vi "Change Qpurge.vi"(8 "error in":errorcluster, 11 "tCRD in":refnum<class "Open Path CRD.lvclass">) -> (0 "error out":errorcluster, 3 "tCRD out":refnum<class "Open Path CRD.lvclass">)   [LabVIEW 2015, in "Open Path CRD.lvclass"]
uses:
  Open Path CRD.lvclass
  Reusable/Instrument/Instrument.lvclass/Instrument.ctl
  Open Path CRD.lvclass/Open Path CRD.ctl
  Reusable/Instrument/Read Log Session.vi
  Reusable/CRDS/Main/Read Data.vi
  Reusable/CRDS/Data/Main/Read filter.vi
  Reusable/CRDS/Data/Main/CRDS Data.lvclass
  <userlib>/_Session Fwk/Session - Root.lvclass
  Devices/Alicat/Session Based/Alicat Device.lvclass
  Reusable/Session Log/System Log.lvclass
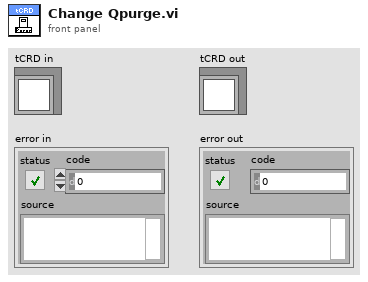
[diagram p1: front panel]
types:
  T1 = typedef "Session - Root.lvclass/Session Handle.ctl" = refnum<data-value>
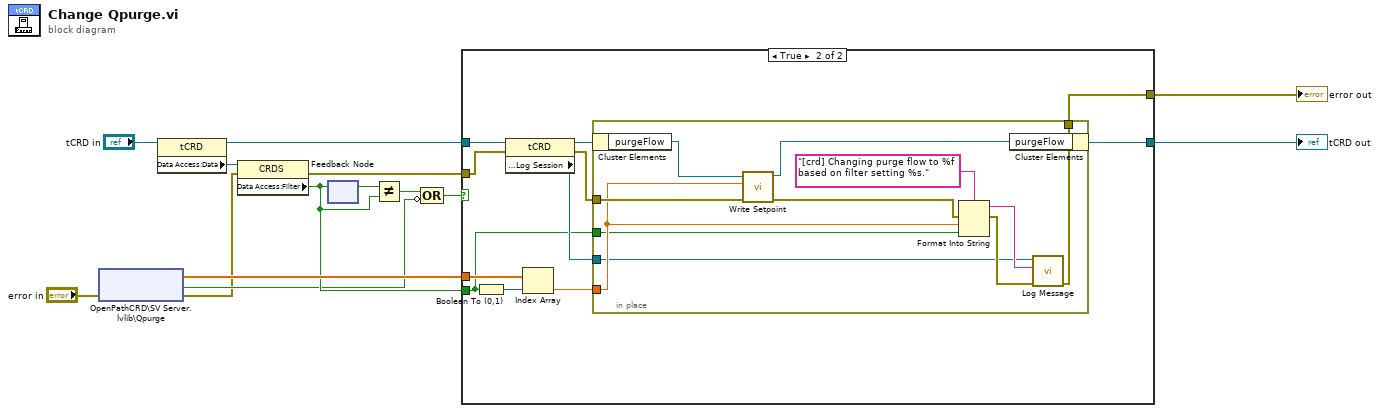
[diagram p0: block diagram]
diagram:
  n1 = shared-variable "OpenPathCRD\\SV Server.lvlib\\Qpurge"(error in="error in") -> (w11:sgl[], error out=w2:errorcluster, w3:bool)  [unwired: 1 in]
  n2 = property class="tCRD"(reference="tCRD in") -> (reference out=w9:refnum<class "Open Path CRD.lvclass">, "Data Access:Data"=w8:refnum<class "CRDS Data.lvclass">)  [unwired: 1 in, 1 out]
  n3 = property class="CRDS"(reference=w8, error in=w2) -> (error out=w1:errorcluster, "Data Access:Filter"=w4:bool)  [unwired: 1 out]
  n4 = feedback-in #1(w4) -> ()
  n5 = feedback #1() -> (w7:bool)  [unwired: 1 in]
  n6 = Not Equal?(x=w7, y=w4) -> (x != y?=w6:bool)
  n7 = Compound Arithmetic op=OR(w6, invert w3) -> (w5:bool)
  n8 = case shown="True" w5 {
    tunnel: w9 -> [w16 w26]
    tunnel: [w16 w27] -> w12
    tunnel: [w15 w24] -> w14
    tunnel: w11 -> [_ w22]
    tunnel: w4 -> [_ w20]
    tunnel: w1 -> [w15 w17]
    frame False {
    }
    frame True {
      n9 = Boolean To (0,1)(Boolean=w20) -> (0, 1=w23:i16)
      n10 = property class="tCRD"(reference=w26, error in=w17) -> (reference out=w19:refnum<class "Open Path CRD.lvclass">, error out=w18:errorcluster, "Accessors:Log Session"=w25:T1)
      n11 = Index Array(array=w22, index=w23) -> (element=w21:sgl)
      n12 = in-place {
        in-place-border: w21 -> [w34]
        in-place-border: w18 -> [w38]
        in-place-border: w25 -> [w30]
        in-place-border: [w29] -> w24
        in-place-border: w20 -> [w28]
        n13 = in-place-cluster #2(w19) -> ("purgeFlow"=w37:refnum<class "Alicat Device.lvclass">)
        n14 = call "Write Setpoint.vi"("error in"=w38, "Setpoint"=w34, "Alicat Device in"=w37) -> ("error out"=w33:errorcluster, "Alicat Device out"=w36:refnum<class "Alicat Device.lvclass">)  [unwired: 6 in, 1 out]
        n15 = Format Into String(format string="[crd] Changing purge flow to %f based on filter setting %s.", error in=w33, w34, w28) -> (resulting string=w31:string, error out=w32:errorcluster)  [unwired: 1 in]
        n16 = in-place-cluster #2("purgeFlow"=w36) -> (w27:refnum<class "Open Path CRD.lvclass">)
        n17 = call "Log Message.vi"("error in"=w32, "MSG In"=w31, "session in"=w30) -> ("error out"=w29:errorcluster)  [unwired: 7 in, 1 out]
      }
    }
  }
  "error out" <- w14
  "tCRD out" <- w12
